vi "AOL Z Cal-Automation module.vi"(9 "Timed out while waiting for acknowledgement in":bool, 10 "FOR loop index":i32, 11 "Initial motor position (um)":sgl) -> (1 "Motor timed out or errored out":bool, 2 "Cancelled":bool, 3 "Measured cal value":sgl)   [LabVIEW 2017]
uses:
  Globals/gl_Calibration globals.vi
panel:
  in  "Max offset (us)":i32=10 min=5 max=100
  in  "Wait before measurement (ms)":u32=500
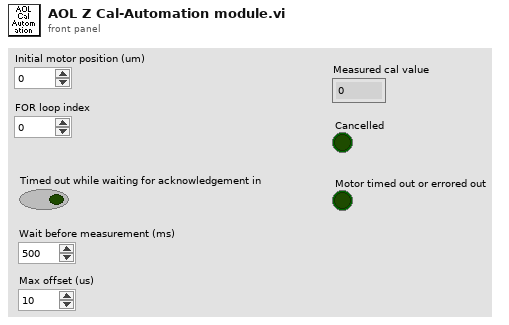
[diagram p1: front panel]
types:
  T1 = typedef "AOL Z cal process refs.ctl" = cluster{"This VI":refnum<vi>, "Abort (ind)":refnum<vi>, "Next (ind)":refnum<vi>, "Cancel":refnum<vi>, "Next":refnum<vi>, "Message":refnum<vi>}
  T2 = typedef "Cal mode.ctl" = enum16{"Automatic", "Interactive"}
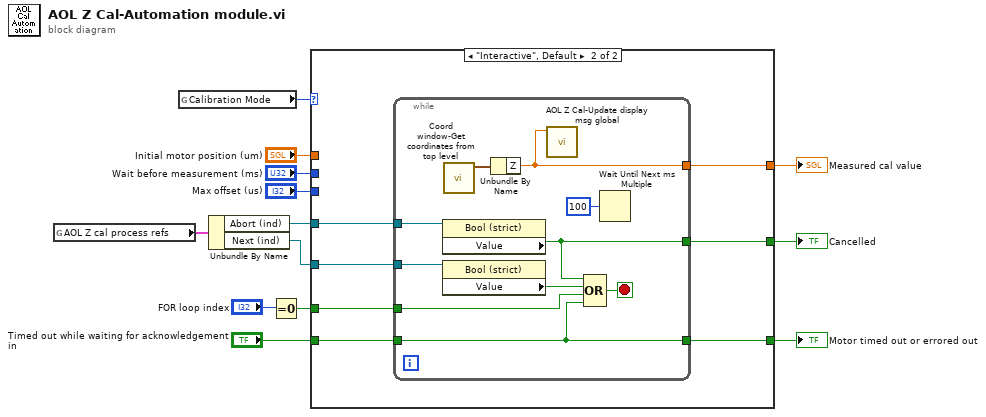
[diagram p0: block diagram]
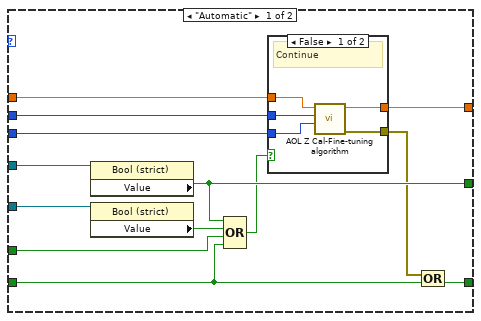
[diagram p2: hidden frame]
diagram:
  n1 = global read "gl_Calibration globals.vi" "AOL Z cal process refs"() -> (w7:T1)
  n2 = global read "gl_Calibration globals.vi" "Calibration Mode"() -> (w1:T2)
  n3 = Unbundle By Name(w7) -> ("Abort (ind)"=w12:refnum<vi>, "Next (ind)"=w13:refnum<vi>)
  n4 = Equal To 0?(x="FOR loop index") -> (x = 0?=w4:bool)
  n5 = case shown="\"Interactive\", Default" w1 {
    tunnel: w13 -> [w26 w38]
    tunnel: w12 -> [w25 w37]
    tunnel: "Initial motor position (um)" -> [w24 _]
    tunnel: [w23 w36] -> w10
    tunnel: "Timed out while waiting for acknowledgement in" -> [w22 w35]
    tunnel: [w21 w34] -> w8
    tunnel: "Wait before measurement (ms)" -> [w20 _]
    tunnel: w4 -> [w19 w33]
    tunnel: [w18 w32] -> w3
    tunnel: "Max offset (us)" -> [w17 _]
    frame "Automatic" {
      n6 = property class="Bool (strict)"(reference=w25) -> ("Value"=w21:bool)  [unwired: 1 in, 2 out]
      n7 = property class="Bool (strict)"(reference=w26) -> ("Value"=w16:bool)  [unwired: 1 in, 2 out]
      n8 = Compound Arithmetic op=OR(w21, w16, w19, w22) -> (w15:bool)
      n9 = case shown="False" w15 {
        tunnel: w24 -> [w31 _]
        tunnel: w20 -> [w30 _]
        tunnel: [w29 _] -> w18
        tunnel: [w28 _] -> w14
        tunnel: w17 -> [w27 _]
        frame False {
          # "Continue"
          n10 = call "AOL Z Cal-Fine-tuning algorithm.vi"("Max offset (us)"=w27, "Wait before measurement (ms)"=w30, "Initial motor position (um)"=w31) -> ("error out"=w28:errorcluster, "Measured cal value"=w29:sgl)  [unwired: 7 in]
        }
        frame True {
          # "Abort"
        }
      }
      n11 = Compound Arithmetic op=OR(w14, w22) -> (w23:bool)
    }
    frame "Interactive", Default {
      n12 = while {
        tunnel: w38 -> [w48]
        tunnel: w37 -> [w47]
        tunnel: [w42] -> w36
        tunnel: w35 -> [w42]
        tunnel: [w46] -> w34
        tunnel: w33 -> [w45]
        tunnel: [w39] -> w32
        stop <- w43 stop-if-true
        n13 = property class="Bool (strict)"(reference=w47) -> ("Value"=w46:bool)  [unwired: 1 in, 2 out]
        n14 = property class="Bool (strict)"(reference=w48) -> ("Value"=w44:bool)  [unwired: 1 in, 2 out]
        n15 = call "Coord window-Get coordinates from top level.vi"() -> ("Coordinates"=w40:cluster{"X":sgl, "Y":sgl, "Z":sgl})  [unwired: 11 in]
        n16 = Unbundle By Name(w40) -> ("Z"=w39:sgl)
        n17 = call "AOL Z Cal-Update display msg global.vi"("Motor Z"=w39) -> ()  [unwired: 11 in]
        n18 = Compound Arithmetic op=OR(w46, w44, w45, w42) -> (w43:bool)
        n19 = Wait Until Next ms Multiple(millisecond multiple=u32 100) -> ()  [unwired: 1 out]
      }
    }
  }
  "Motor timed out or errored out" <- w10
  "Cancelled" <- w8
  "Measured cal value" <- w3
